vi "Interface.vi"() -> ()   [LabVIEW 2019]
uses:
  <vilib>/numeric/Random Number (Range) I64.vi
  <vilib>/numeric/sub_Random U32.vi
panel:
  in  "ArrayForChart":i32[](array[numeric])
  in  "StartBlinkingCounter":u32
  out "current time":timestamp
  in  "MainTab":enum32{"Homepage", "Graph", "File IO", "About"}(tab)
  out "BlinkingLED":bool
  in  "StartBlinking":bool
  out "NumericMouseDetector":bool
  out "NumericChangeDetector":bool
  in  "NumericToControl":i32
  in  "GetCurrentTime":bool
  out "current time with button":timestamp
  out "OldVal":i32
  out "NewVal":i32
  out "Waveform Graph":dbl[](graph)
  in  "OnOffData":bool
  in  "WriteAppend":bool
  in  "WriteNew":bool
  in  "Content":string
  in  "File Title":string
  out "error out":errorcluster
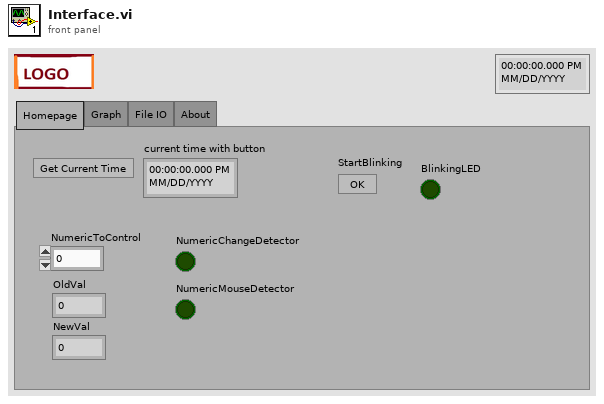
[diagram p1: front panel]
types:
  T1 = enum16{"open", "replace", "create", "open or create", "replace or create", "replace or create with confirmation"}
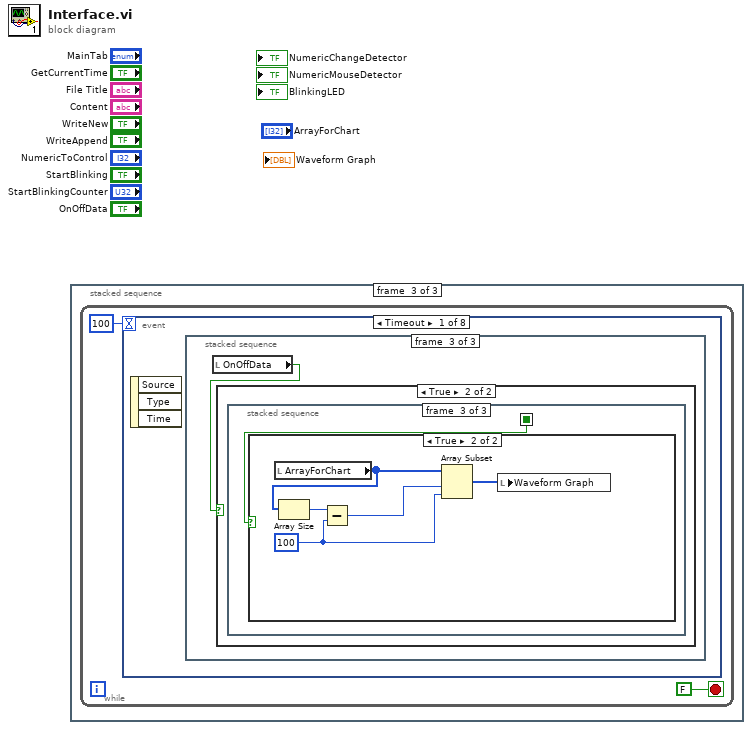
[diagram p0: block diagram]
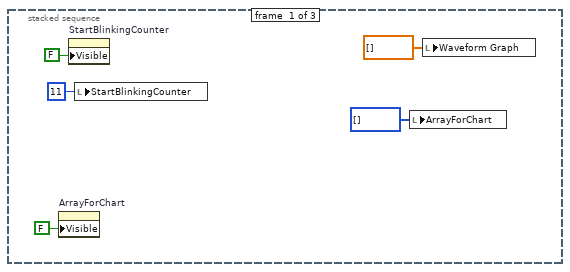
[diagram p2: hidden frame]
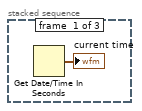
[diagram p4: hidden frame]
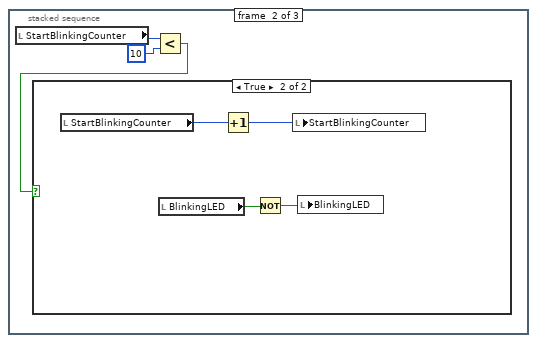
[diagram p5: hidden frame]
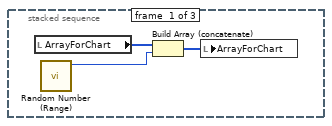
[diagram p8: hidden frame]
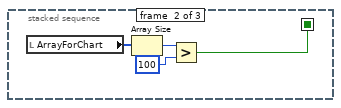
[diagram p9: hidden frame]
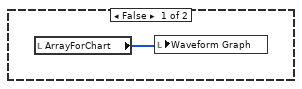
[diagram p10: hidden frame]
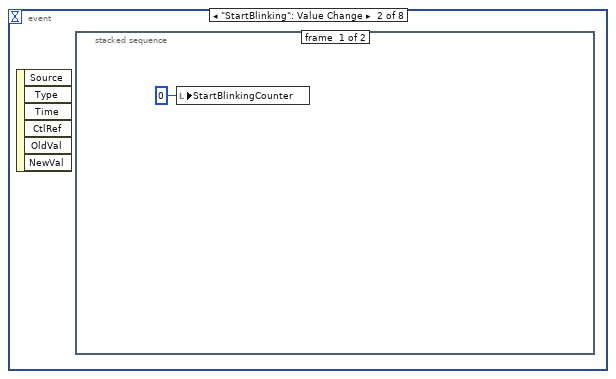
[diagram p11: hidden frame]
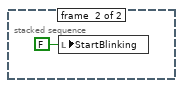
[diagram p12: hidden frame]
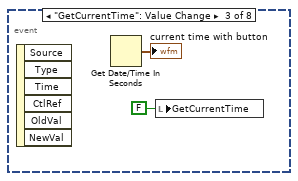
[diagram p13: hidden frame]
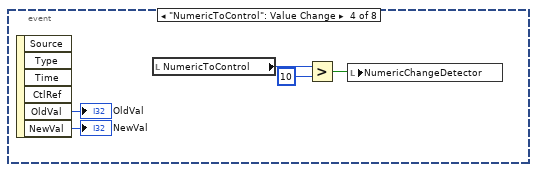
[diagram p14: hidden frame]
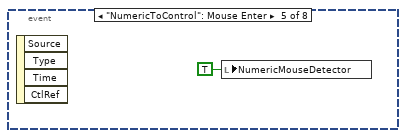
[diagram p15: hidden frame]
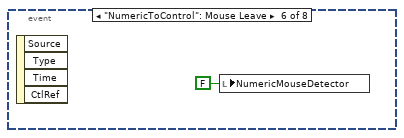
[diagram p16: hidden frame]
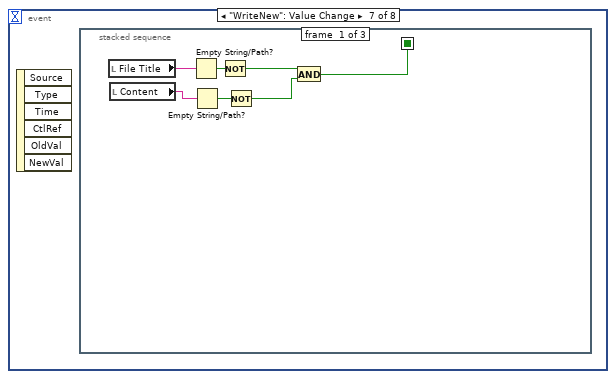
[diagram p17: hidden frame]
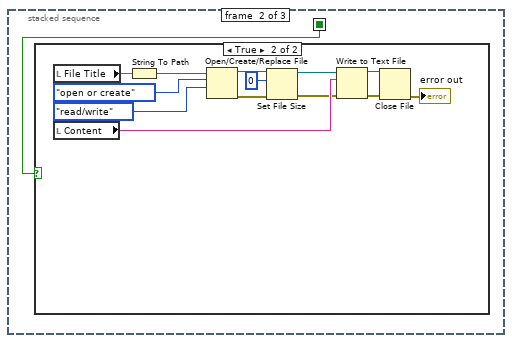
[diagram p18: hidden frame]
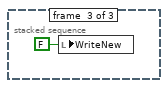
[diagram p20: hidden frame]
diagram:
  n1 = stacked-sequence {
    frame #0 {
      n2 = property on="ArrayForChart" class="Arr (strict)"("Visible"=FALSE) -> ()  [unwired: 2 in, 2 out]
      n3 = property on="StartBlinkingCounter" class="DigNum (strict)"("Visible"=FALSE) -> ()  [unwired: 2 in, 2 out]
      n4 = local write "StartBlinkingCounter"(u32 11 ("StartBlinkingCounter")) -> ()
      n5 = local write "ArrayForChart"(i32[] [] ("ArrayForChart")) -> ()
      n6 = local write "Waveform Graph"(dbl[] [] ("Waveform Graph")) -> ()
    }
    frame #1 {
    }
    frame #2 {
      n7 = while {
        stop <- FALSE stop-if-true
        n8 = event shown="[0] Timeout" {
          selector: _ -> [_ _ _ _ _ _ _ _]
          dyn-events: _ -> [_ _ _ _ _ _ _ _]
          timeout: 100 -> [_ _ _ _ _ _ _ _]
          event Timeout {
            n9 = event-data() -> ()  [unwired: 1 in, 3 out]
            n10 = stacked-sequence {
              frame #0 {
                n11 = Get Date/Time In Seconds() -> (seconds since 1Jan1904=→"current time":timestamp)
              }
              frame #1 {
                n12 = local read "StartBlinkingCounter"() -> (w11:u32)
                n13 = Less?(x=w11, y=u32 10) -> (x < y?=w9:bool)
                n14 = case shown="True" w9 {
                  frame False {
                  }
                  frame True {
                    n15 = local read "StartBlinkingCounter"() -> (w15:u32)
                    n16 = local read "BlinkingLED"() -> (w12:bool)
                    n17 = Increment(x=w15) -> (x+1=w14:u32)
                    n18 = Not(x=w12) -> (.not. x?=w13:bool)
                    n19 = local write "StartBlinkingCounter"(w14) -> ()
                    n20 = local write "BlinkingLED"(w13) -> ()
                  }
                }
              }
              frame #2 {
                n21 = local read "OnOffData"() -> (w16:bool)
                n22 = case shown="True" w16 {
                  frame False {
                  }
                  frame True {
                    n23 = stacked-sequence {
                      seq-local: [_ w20 _] -> [_ _ w24]
                      frame #0 {
                        n24 = local read "ArrayForChart"() -> (w19:i32[])
                        n25 = call-poly <vilib>:"Random Number (Range).vi"() -> ("number"=w18:i64)  [unwired: 11 in]
                        n26 = Build Array (concatenate)(w19, w18) -> (w17:i64[])
                        n27 = local write "ArrayForChart"(w17) -> ()
                      }
                      frame #1 {
                        n28 = local read "ArrayForChart"() -> (w23:i32[])
                        n29 = Array Size(array=w23) -> (size(s)=w22:i32)
                        n30 = Greater?(x=w22, y=100) -> (0:w20:bool)
                      }
                      frame #2 {
                        n31 = case shown="True" w24 {
                          frame False {
                            n32 = local read "ArrayForChart"() -> (w25:i32[])
                            n33 = local write "Waveform Graph"(w25) -> ()
                          }
                          frame True {
                            w28 = 100 ("length")
                            n34 = local read "ArrayForChart"() -> (w30:i32[])
                            n35 = Array Size(array=w30) -> (size(s)=w29:i32)
                            n36 = Subtract(x=w29, y=w28) -> (x-y=w27:i32)
                            n37 = Array Subset(array=w30, index=w27, length=w28) -> (w26:i32[])
                            n38 = local write "Waveform Graph"(w26) -> ()
                          }
                        }
                      }
                    }
                  }
                }
              }
            }
          }
          event "StartBlinking": Value Change {
            n39 = event-data() -> ()  [unwired: 1 in, 6 out]
            n40 = stacked-sequence {
              frame #0 {
                n41 = local write "StartBlinkingCounter"(u32 0 ("StartBlinkingCounter")) -> ()
              }
              frame #1 {
                n42 = local write "StartBlinking"(FALSE ("StartBlinking")) -> ()
              }
            }
          }
          event "GetCurrentTime": Value Change {
            n43 = event-data() -> ()  [unwired: 1 in, 6 out]
            n44 = Get Date/Time In Seconds() -> (seconds since 1Jan1904=→"current time with button":timestamp)
            n45 = local write "GetCurrentTime"(FALSE ("GetCurrentTime")) -> ()
          }
          event "NumericToControl": Value Change {
            n46 = event-data() -> ("OldVal"=→"OldVal":i32, "NewVal"=→"NewVal":i32)  [unwired: 1 in, 4 out]
            n47 = local read "NumericToControl"() -> (w39:i32)
            n48 = Greater?(x=w39, y=10) -> (0:w37:bool)
            n49 = local write "NumericChangeDetector"(w37) -> ()
          }
          event "NumericToControl": Mouse Enter {
            n50 = event-data() -> ()  [unwired: 1 in, 4 out]
            n51 = local write "NumericMouseDetector"(TRUE ("NumericMouseDetector")) -> ()
          }
          event "NumericToControl": Mouse Leave {
            n52 = event-data() -> ()  [unwired: 1 in, 4 out]
            n53 = local write "NumericMouseDetector"(FALSE ("NumericMouseDetector")) -> ()
          }
          event "WriteNew": Value Change {
            n54 = event-data() -> ()  [unwired: 1 in, 6 out]
            n55 = stacked-sequence {
              seq-local: [w48 _ _] -> [_ w49 _]
              frame #0 {
                n56 = local read "File Title"() -> (w47:string)
                n57 = local read "Content"() -> (w46:string)
                n58 = Empty String/Path?(string/path=w47) -> (empty?=w45:bool)
                n59 = Empty String/Path?(string/path=w46) -> (empty?=w44:bool)
                n60 = Not(x=w45) -> (.not. x?=w43:bool)
                n61 = Not(x=w44) -> (.not. x?=w42:bool)
                n62 = And(x=w43, y=w42) -> (x .and. y?=w48:bool)
              }
              frame #1 {
                n63 = case shown="True" w49 {
                  frame False {
                  }
                  frame True {
                    n64 = local read "File Title"() -> (w62:string)
                    n65 = local read "Content"() -> (w58:string)
                    n66 = String To Path(string=w62) -> (path=w61:path)
                    n67 = Open/Create/Replace File(file path (use dialog)=w61, operation (0:open)=T1."open or create", access (0:read/write)=enum16{"read/write", "read-only", "write-only"}."read/write") -> (refnum out=w54:refnum<file>, error out=w51:errorcluster)  [unwired: 3 in, 1 out]
                    n68 = Set File Size(4:w51, 6:i64 0 ("size (in bytes)"), 7:w54) -> (0:w52:errorcluster, 3:w53:refnum<file>)
                    n69 = Write to Text File(file (use dialog)=w53, text=w58, error in=w52) -> (refnum out=w56:refnum<file>, error out=w57:errorcluster)  [unwired: 1 in, 1 out]
                    n70 = Close File(refnum=w56, error in=w57) -> (error out=→"error out":errorcluster)  [unwired: 1 out]
                  }
                }
              }
              frame #2 {
                n71 = local write "WriteNew"(FALSE ("WriteNew")) -> ()
              }
            }
          }
          event "WriteAppend": Value Change {
            n72 = event-data() -> ()  [unwired: 1 in, 6 out]
            n73 = stacked-sequence {
              seq-local: [w64 _ _] -> [_ w72 _]
              frame #0 {
                w67 = 0 ("y")
                n74 = local read "File Title"() -> (w71:string)
                n75 = local read "Content"() -> (w70:string)
                n76 = String Length(string=w70) -> (length=w68:i32)
                n77 = String Length(string=w71) -> (length=w69:i32)
                n78 = Not Equal?(x=w69, y=w67) -> (x != y?=w66:bool)
                n79 = Not Equal?(x=w68, y=w67) -> (x != y?=w65:bool)
                n80 = And(x=w66, y=w65) -> (x .and. y?=w64:bool)
              }
              frame #1 {
                n81 = case shown="True" w72 {
                  frame False {
                  }
                  frame True {
                    n82 = local read "File Title"() -> (w84:string)
                    n83 = local read "Content"() -> (w82:string)
                    n84 = String To Path(string=w84) -> (path=w83:path)
                    n85 = Open/Create/Replace File(file path (use dialog)=w83, operation (0:open)=T1."open or create", access (0:read/write)=enum16{"read/write", "read-only", "write-only"}."read/write") -> (refnum out=w77:refnum<file>, error out=w76:errorcluster)  [unwired: 3 in, 1 out]
                    n86 = Set File Position(refnum=w77, from (0:start)=enum16{"start", "end", "current"}."end", error in=w76) -> (refnum out=w75:refnum<file>, error out=w74:errorcluster)  [unwired: 1 in]
                    n87 = Write to Text File(file (use dialog)=w75, text=w82, error in=w74) -> (refnum out=w80:refnum<file>, error out=w81:errorcluster)  [unwired: 1 in, 1 out]
                    n88 = Close File(refnum=w80, error in=w81) -> (error out=w85:errorcluster)  [unwired: 1 out]
                    n89 = local write "error out"(w85) -> ()
                  }
                }
              }
              frame #2 {
                n90 = local write "WriteAppend"(FALSE ("WriteAppend")) -> ()
              }
            }
          }
        }
      }
    }
  }
